vi "NATS Client stop.vi"(8 "error in":errorcluster, 11 "NATS Client":refnum<class "NATS Client.lvclass">) -> (0 "error out":errorcluster)   [LabVIEW 2024, in "NATS Client.lvlib" / "NATS Client.lvclass"]
doc: "Reads a message from the NATS server."
uses:
  NATS Client.lvclass
  NATS Client.lvclass/NATS Client.ctl
  NATS Core.lvlib
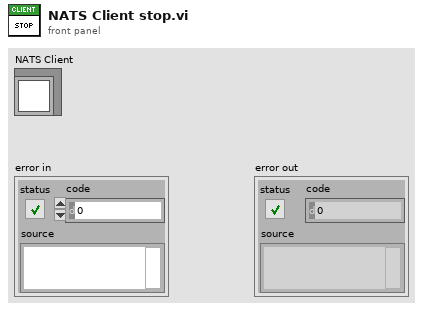
[diagram p1: front panel]
types:
  T1 = typedef "NATS Core.lvlib/nats connection.ctl" = cluster{"connection ID":refnum<k5>, "server INFO":string, "timeout ms":i32, "verbose?":bool, "server headers?":bool, "client headers?":bool}
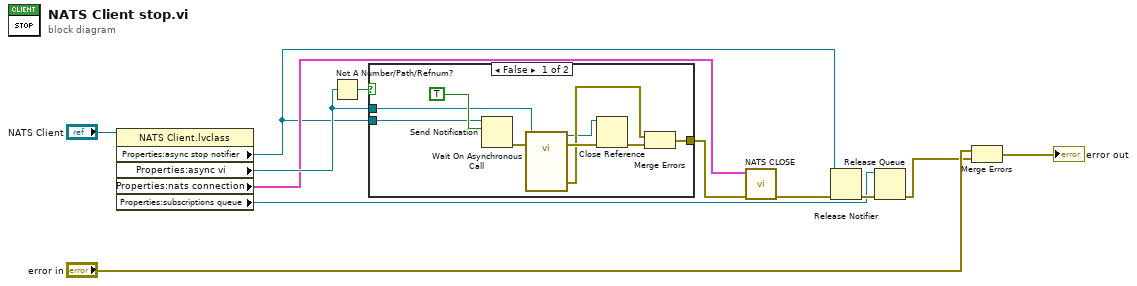
[diagram p0: block diagram]
diagram:
  n1 = property class="NATS Client.lvclass"(reference="NATS Client") -> ("Properties:async stop notifier"=w1:refnum<notifier>, "Properties:async vi"=w4:refnum<vi>, "Properties:nats connection"=w2:T1, "Properties:subscriptions queue"=w3:refnum<queue>)  [unwired: 1 in, 2 out]
  n2 = Not A Number/Path/Refnum?(number/path/refnum=w4) -> (NaN/Path/Refnum?=w6:bool)
  n3 = case shown="False" w6 {
    tunnel: [w19 _] -> w8
    tunnel: w4 -> [w14 _]
    tunnel: w1 -> [w13 _]
    frame False {
      n4 = Send Notification(notification=TRUE, notifier=w13) -> (error out=w20:errorcluster)  [unwired: 1 in, 1 out]
      n5 = call-by-ref "Wait On Asynchronous Call"(reference=w14, error in=w20) -> (reference out=w15:refnum<vi>, error out=w21:errorcluster, 0:"error out"=w18:errorcluster)  [unwired: 11 in]
      n6 = Close Reference(reference=w15, error in (no error)=w21) -> (error out=w17:errorcluster)
      n7 = Merge Errors(w18, w17) -> (w19:errorcluster)
    }
    frame True {
    }
  }
  n8 = call "NATS CLOSE.vi"("error in"=w8, "nats connection in"=w2) -> ("error out"=w7:errorcluster)  [unwired: 9 in]
  n9 = Release Notifier(notifier=w1, error in (no error)=w7) -> (error out=w10:errorcluster)  [unwired: 1 in, 2 out]
  n10 = Release Queue(queue=w3, error in (no error)=w10) -> (error out=w9:errorcluster)  [unwired: 1 in, 2 out]
  n11 = Merge Errors("error in", w9) -> (→"error out":errorcluster)
